vi "Unique_Selector_Values.vi"(2 "Number that means blank":dbl=60221366999.69 format="%#.3f", 3 "Precision":string, 4 "Bin Centres":dbl[](array[numeric]) format="%.4f") -> (1 "Bin Strings":string[](array[string]))   [LabVIEW 2010]
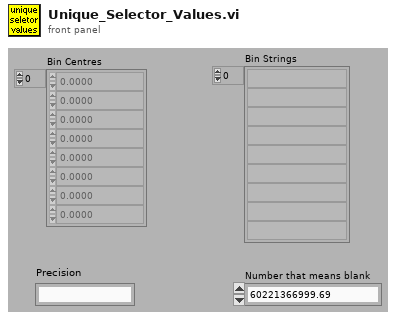
[diagram p1: front panel]
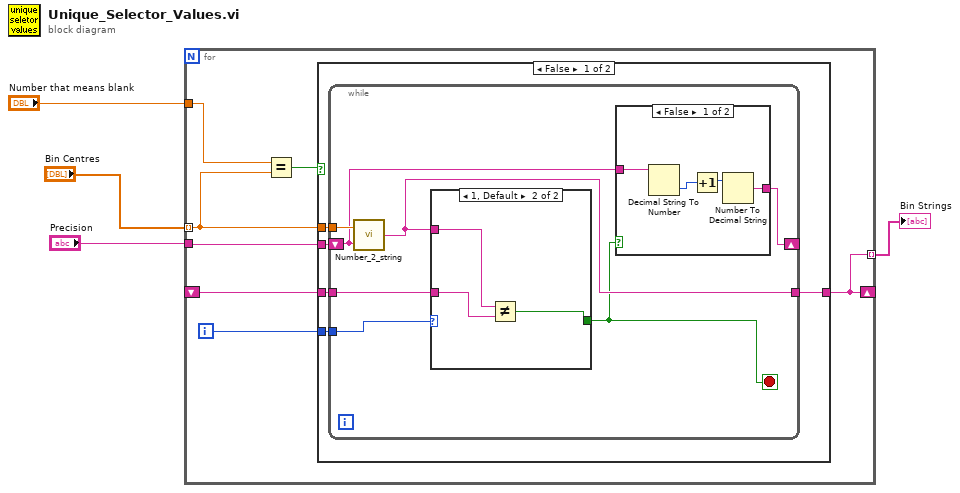
[diagram p0: block diagram]
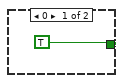
[diagram p3: hidden frame]
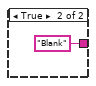
[diagram p4: hidden frame]
diagram:
  n1 = for {
    tunnel: "Bin Centres" -> [w6] mode=indexing
    tunnel: "Precision" -> [w9]
    shift-right: [w8] -> _
    shift-left: _ -> [w10]
    tunnel: [w8] -> w2 mode=indexing
    tunnel: "Number that means blank" -> [w5]
    i -> [w11]
    n2 = Equal?(x=w5, y=w6) -> (x = y?=w7:bool)
    n3 = case shown="False" w7 {
      tunnel: w6 -> [w16 _]
      tunnel: w11 -> [w15 _]
      tunnel: w10 -> [w14 _]
      tunnel: w9 -> [w13 _]
      tunnel: [w12 "Blank" ("String")] -> w8
      frame False {
        n4 = while {
          tunnel: w16 -> [w23]
          tunnel: w15 -> [w22]
          tunnel: w14 -> [w21]
          tunnel: [w20] -> w12
          shift-right: [w17] -> _
          shift-left: w13 -> [w18]
          stop <- w19 stop-if-true
          n5 = call "Number_2_string.vi"("precision"=w18, "number"=w23) -> ("String"=w20:string)
          n6 = case shown="1, Default" w22 {
            tunnel: w20 -> [_ w32]
            tunnel: w21 -> [_ w31]
            tunnel: [TRUE w30] -> w19
            frame 0 {
            }
            frame 1, Default {
              n7 = Not Equal?(x=w32, y=w31) -> (x != y?=w30:bool)
            }
          }
          n8 = case shown="False" w19 {
            tunnel: w18 -> [w27 w28]
            tunnel: [w24 w28] -> w17
            frame False {
              n9 = Decimal String To Number(string=w27) -> (number=w26:i32)  [unwired: 3 out]
              n10 = Increment(x=w26) -> (x+1=w25:i32)
              n11 = Number To Decimal String(number=w25) -> (decimal integer string=w24:string)  [unwired: 1 out]
            }
            frame True {
            }
          }
        }
      }
      frame True {
      }
    }
  }
  "Bin Strings" <- w2
